vi "Read Tag.vi"(0 "ignore previous (F)":bool, 2 "EnclaveChannel":T2, 3 "timeout in ms (-1)":i32=-1) -> (1 "Time Stamp":timestamp, 5 "New Value?":bool, 7 "Element":T1, 8 "Closed?":bool, 9 "timed out?":bool)   [LabVIEW 2022 SP3, in "Enclave.lvlib"]
doc: "Reads the latest value from the Channel Wire. The endpoint can optionally be configured to wait for a new value by setting <b>ignore previous</b> to true."
uses:
  Enclave.lvlib
  ))Channel.ctl
  Element.ctl
  Tag/Tag.lvclass
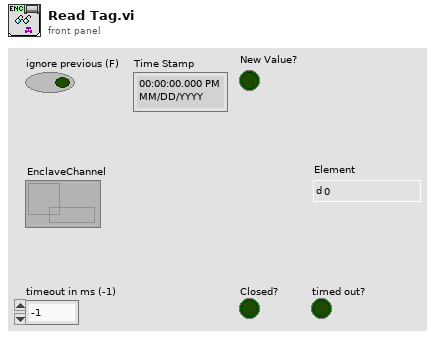
[diagram p1: front panel]
types:
  T1 = typedef "Enclave.lvlib/Element.ctl" = dbl
  T2 = typedef "Enclave.lvlib/))Channel.ctl" = refnum<queue>
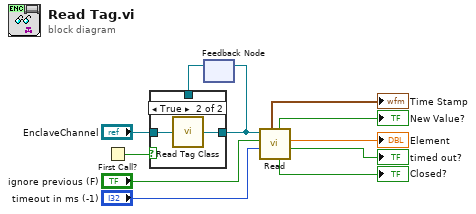
[diagram p0: block diagram]
diagram:
  n1 = First Call?() -> (First Call?: T/F=w10:bool)
  n2 = feedback #1() -> (w5:refnum<class "Tag.lvclass">)  [unwired: 1 in]
  n3 = case shown="True" w10 {
    tunnel: "EnclaveChannel" -> [_ w14]
    tunnel: [w12 w13] -> w4
    tunnel: w5 -> [w12 _]
    frame False {
    }
    frame True {
      n4 = call "Read Tag Class.vi"("EnclaveChannel"=w14) -> ("Lossy Reader"=w13:refnum<class "Tag.lvclass">)  [unwired: 7 in, 1 out]
    }
  }
  n5 = feedback-in #1(w4) -> ()
  n6 = call "Read.vi"("timeout in ms (-1)"="timeout in ms (-1)", "ignore previous (F)"="ignore previous (F)", "Tag in"=w4) -> ("timed out?"=→"timed out?":bool, "Element"=→"Element":T1, "Closed?"=→"Closed?":bool, "New Value?"=→"New Value?":bool, "Time Stamp"=→"Time Stamp":timestamp)  [unwired: 4 in]
